vi "Read Module Status.vi"(8 "error in":errorcluster, 11 "Module Editor Node in":refnum<class "module editor node.lvclass">) -> (0 "error out":errorcluster, 2 "module status":T1, 3 "Module Editor Node out":refnum<class "module editor node.lvclass">)   [LabVIEW 2013, in "PL Framework Configuration Tool.lvlib" / "module editor node.lvclass"]
uses:
  module editor node.lvclass
  subVIs/Glyphs Status.ctl
  <vilib>/NI/Tag Bus Module Framework/module configuration/TBM module configuration.lvclass
  Read Module Configuration.vi
  PL Framework Configuration Tool.lvlib
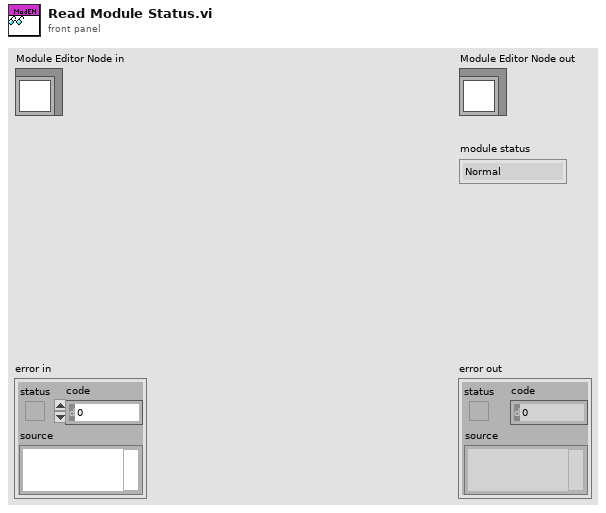
[diagram p1: front panel]
types:
  T1 = typedef "PL Framework Configuration Tool.lvlib/Glyphs Status.ctl" = enum16{"Normal", "Error"}
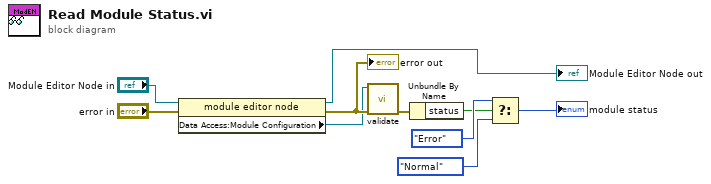
[diagram p0: block diagram]
diagram:
  n1 = property class="module editor node"(reference="Module Editor Node in", error in="error in") -> (reference out=→"Module Editor Node out":refnum<class "module editor node.lvclass">, error out=w4:errorcluster, "Data Access:Module Configuration"=w3:refnum<class "TBM module configuration.lvclass">)
  "error out" <- w4
  n2 = call-dynamic "validate.vi"("error in"=w4, "configuration in"=w3) -> ("error out"=w2:errorcluster)  [unwired: 8 in, 1 out]
  n3 = Unbundle By Name(w2) -> ("status"=w1:bool)
  n4 = Select(t=Glyphs_Status."Error", s=w1, f=Glyphs_Status."Normal" ("component status")) -> (s? t:f=→"module status":T1)
